vi "Queue In Free.vi"(7 "First":bool, 8 "error in (no error)":errorcluster caption="Error In", 9 "Data":variant, 10 "Message":string, 11 "Queue In":refnum<queue>) -> (0 "error out":errorcluster caption="Error Out", 3 "Queue Out":refnum<queue>)   [LabVIEW 2020]
uses:
  Queue Message.ctl
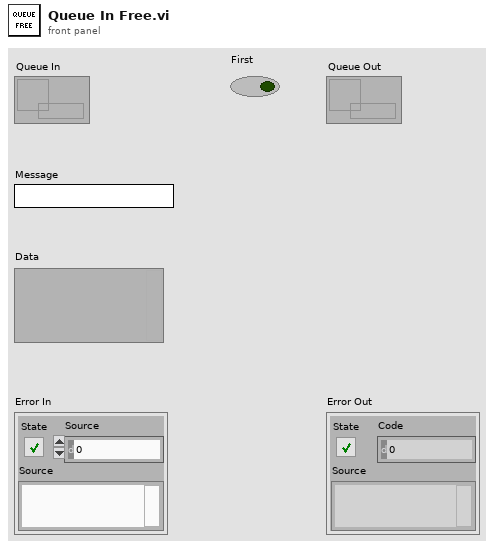
[diagram p1: front panel]
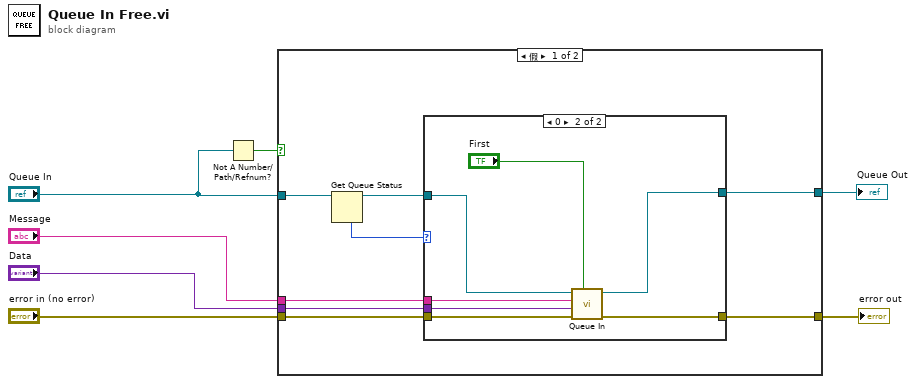
[diagram p0: block diagram]
diagram:
  n1 = Not A Number/Path/Refnum?(number/path/refnum="Queue In") -> (NaN/Path/Refnum?=w1:bool)
  n2 = case shown="假" w1 {
    tunnel: "error in (no error)" -> [w15 w25]
    tunnel: "Data" -> [w14 _]
    tunnel: "Message" -> [w13 _]
    tunnel: [w12 w25] -> w4
    tunnel: [w11 w26] -> w3
    tunnel: "Queue In" -> [w8 w26]
    frame False {
      n3 = Get Queue Status(queue=w8) -> (queue out=w9:refnum<queue>, # elements in queue=w10:i32)  [unwired: 2 in, 6 out]
      n4 = case shown="0" w10 {
        tunnel: w15 -> [w16 w24]
        tunnel: w14 -> [_ w23]
        tunnel: w13 -> [_ w22]
        tunnel: [w16 w21] -> w12
        tunnel: [w17 w20] -> w11
        tunnel: w9 -> [w17 w19]
        frame 1, Default {
        }
        frame 0 {
          n5 = call "Queue In.vi"("First"="First", "error in (no error)"=w24, "Data"=w23, "Message"=w22, "Queue In"=w19) -> ("error out"=w21:errorcluster, "Queue Out"=w20:refnum<queue>)  [unwired: 5 in]
        }
      }
    }
    frame True {
    }
  }
  "error out" <- w4
  "Queue Out" <- w3
